vi "mupGetLastError.vi"(8 "error in (no error)":errorcluster, 11 "hParser in":u64) -> (0 "error out":errorcluster, 2 "error details":T1, 3 "hParser out":u64)   [LabVIEW 2018, in "mupLib.lvlib"]
doc: "Read error details from muparser. If no error has previously occured, error code and error position will be -1."
uses:
  mupLib.lvlib
  libmuparser-lv.dll
panel:
  # "Read error details from muparser. If no error has previously occured, error code and\nerror position will be -1."
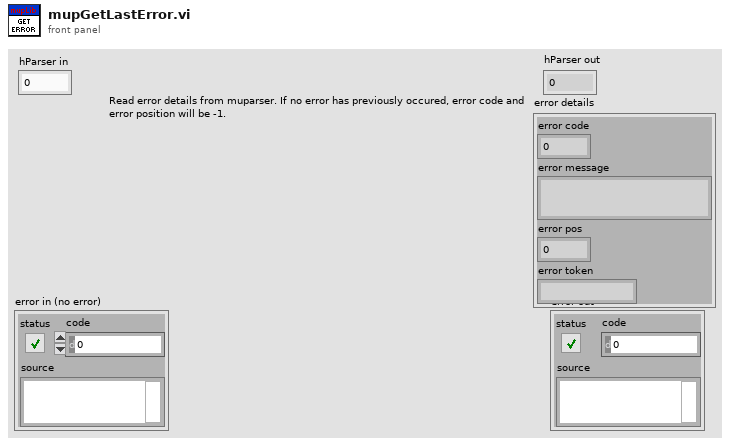
[diagram p1: front panel]
types:
  T1 = cluster{"error code":i32, "error message":string, "error pos":i32, "error token":string}
  T2 = cluster{"error flag":i32, "error message":string, "error pos":i32, "error token":string}
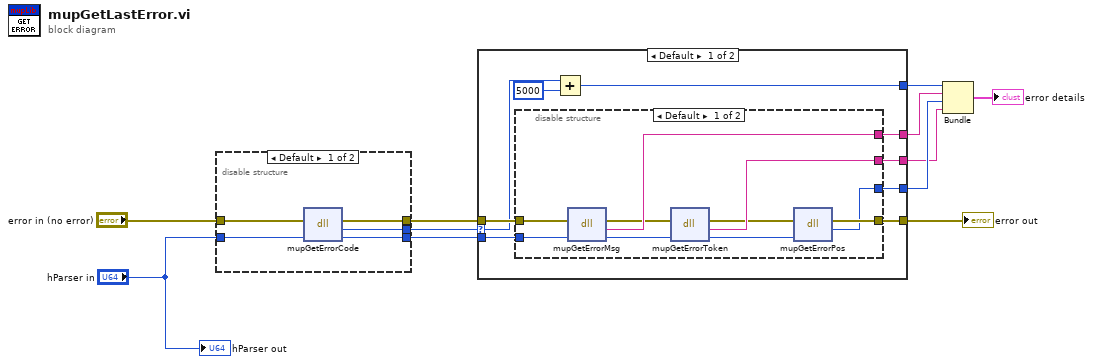
[diagram p0: block diagram]
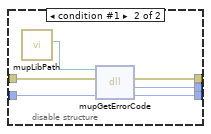
[diagram p2: hidden frame]
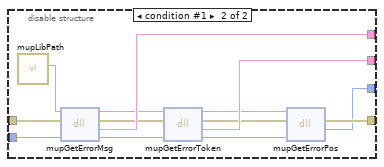
[diagram p3: hidden frame]
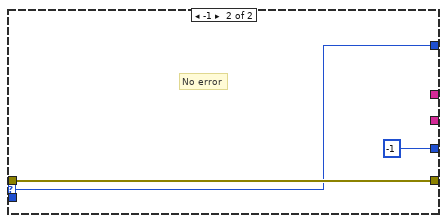
[diagram p4: hidden frame]
diagram:
  n1 = disable-structure shown="Default" {
    disable-tunnel: "error in (no error)" -> [w16 w22]
    disable-tunnel: "hParser in" -> [w15 w21]
    disable-tunnel: [w14 w20] -> w9
    disable-tunnel: [w13 w19] -> w8
    disable-tunnel: [w12 w18] -> w6
    frame condition #0 (active) {
      n2 = dll-call lib="C:/Users/leonidas/Documents/GitHub/LV-muParser/mupLib/libmuparser-lv.dll" fn="mupGetErrorCode"(error in=w16, "hParser"=w15) -> (error out=w14:errorcluster, "error flag"=w12:i32, "hParser"=w13:u64)  [unwired: 2 in, 1 out]
    }
    frame condition #1 {
      n3 = call "mupLibPath.vi"() -> ("libmuparser path"=w17:path)  [unwired: 11 in]
      n4 = dll-call lib="C:/Users/leonidas/Documents/GitHub/LV-muParser/mupLib/libmuparser-lv.dll" fn="mupGetErrorCode"(path in=w17, error in=w22, "hParser"=w21) -> (error out=w20:errorcluster, "error flag"=w18:i32, "hParser"=w19:u64)  [unwired: 1 in, 1 out]
    }
  }
  n5 = case shown="Default" w6 {
    selector: w6 -> [w25 w55]
    tunnel: w9 -> [w28 w57]
    tunnel: w8 -> [w31 _]
    tunnel: [w30 _] -> w4
    tunnel: [w29 _] -> w2
    tunnel: [w27 w57] -> w7
    tunnel: [w26 -1 ("error pos")] -> w3
    tunnel: [w23 w55] -> w5
    frame Default {
      n6 = disable-structure shown="Default" {
        disable-tunnel: w31 -> [w41 w54]
        disable-tunnel: [w40 w53] -> w30
        disable-tunnel: [w38 w51] -> w29
        disable-tunnel: w28 -> [w37 w50]
        disable-tunnel: [w34 w47] -> w27
        disable-tunnel: [w33 w46] -> w26
        frame condition #0 (active) {
          n7 = dll-call lib="C:/Users/leonidas/Documents/GitHub/LV-muParser/mupLib/libmuparser-lv.dll" fn="mupGetErrorMsg"(error in=w37, "hParser"=w41) -> (error out=w36:errorcluster, "error message"=w40:string, "hParser"=w39:u64)  [unwired: 2 in, 1 out]
          n8 = dll-call lib="C:/Users/leonidas/Documents/GitHub/LV-muParser/mupLib/libmuparser-lv.dll" fn="mupGetErrorToken"(error in=w36, "hParser"=w39) -> (error out=w35:errorcluster, "error token"=w38:string, "hParser"=w32:u64)  [unwired: 2 in, 1 out]
          n9 = dll-call lib="C:/Users/leonidas/Documents/GitHub/LV-muParser/mupLib/libmuparser-lv.dll" fn="mupGetErrorPos"(error in=w35, "hParser"=w32) -> (error out=w34:errorcluster, "error pos"=w33:i32)  [unwired: 3 in, 1 out]
        }
        frame condition #1 {
          n10 = call "mupLibPath.vi"() -> ("libmuparser path"=w44:path)  [unwired: 11 in]
          n11 = dll-call lib="C:/Users/leonidas/Documents/GitHub/LV-muParser/mupLib/libmuparser-lv.dll" fn="mupGetErrorMsg"(path in=w44, error in=w50, "hParser"=w54) -> (path out=w43:path, error out=w49:errorcluster, "error message"=w53:string, "hParser"=w52:u64)  [unwired: 1 in]
          n12 = dll-call lib="C:/Users/leonidas/Documents/GitHub/LV-muParser/mupLib/libmuparser-lv.dll" fn="mupGetErrorToken"(path in=w43, error in=w49, "hParser"=w52) -> (path out=w42:path, error out=w48:errorcluster, "error token"=w51:string, "hParser"=w45:u64)  [unwired: 1 in]
          n13 = dll-call lib="C:/Users/leonidas/Documents/GitHub/LV-muParser/mupLib/libmuparser-lv.dll" fn="mupGetErrorPos"(path in=w42, error in=w48, "hParser"=w45) -> (error out=w47:errorcluster, "error pos"=w46:i32)  [unwired: 2 in, 1 out]
        }
      }
      n14 = Add(x=w25, y=5000) -> (x+y=w23:i32)
    }
    frame -1 {
      # "No error"
    }
  }
  "error out" <- w7
  n15 = Bundle("error flag"=w5, "error message"=w4, "error pos"=w3, "error token"=w2) -> (→"error details":T2)  [unwired: 1 in]
  "hParser out" <- "hParser in"
